vi "When Read U32.vi"(0 "error out":errorcluster, 1 "value":u32, 11 "Configuration In":refnum<class "Mock Configuration.lvclass">) -> (3 "Configuration Out":refnum<class "Mock Configuration.lvclass">)   [LabVIEW 2020, in "Mock Configuration.lvclass"]
doc: "High-level function for reading configuration file data from process class. If the specified key is not present, it is added with the configured default value."
uses:
  Mock Configuration.lvclass
  Mock Configuration.lvclass/Mock Configuration.ctl
  <vilib>/Astemes/LMock/Mock.lvclass
  C:/Program Files (x86)/National Instruments/LabVIEW 2020/vi.lib/Astemes/LMock/Mock.lvclass
  C:/git/danfoss-excel-report-teststand-plugin/tests/Mock Configuration/Mock Configuration.lvclass
  C:/git/danfoss-excel-report-teststand-plugin/source/TestStand Public/Components/Models/ModelPlugin/Astemes_CSVReportGenerator/Configuration/Configuration.lvclass
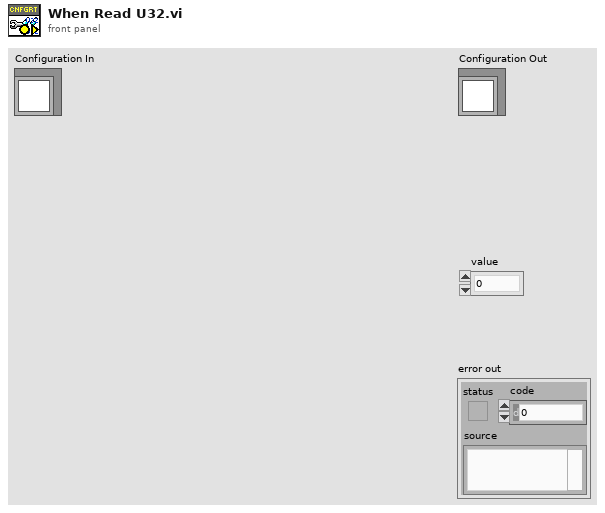
[diagram p1: front panel]
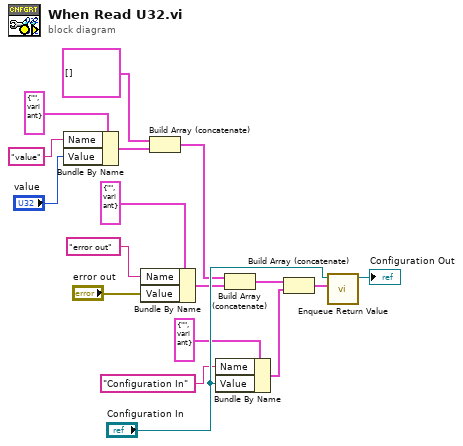
[diagram p0: block diagram]
diagram:
  n1 = Bundle By Name(cluster=cluster{"Name":string, "Value":variant} {"Name"="", "Value"=variant} ("element"), "Name"="value", "Value"="value") -> (w5:cluster{"Name":string, "Value":variant})
  n2 = Bundle By Name(cluster=cluster{"Name":string, "Value":variant} {"Name"="", "Value"=variant} ("element"), "Name"="error out", "Value"="error out") -> (w3:cluster{"Name":string, "Value":variant})
  n3 = Build Array (concatenate)(cluster{"Name":string, "Value":variant}[] [] ("Control Values"), w5) -> (w10:cluster{"Name":string, "Value":variant}[])
  n4 = Bundle By Name(cluster=cluster{"Name":string, "Value":variant} {"Name"="", "Value"=variant} ("element"), "Name"="Configuration In", "Value"="Configuration In") -> (w1:cluster{"Name":string, "Value":variant})
  n5 = Build Array (concatenate)(w10, w3) -> (w13:cluster{"Name":string, "Value":variant}[])
  n6 = Build Array (concatenate)(w13, w1) -> (w15:cluster{"Name":string, "Value":variant}[])
  n7 = call <vilib>:"Enqueue Return Value.vi"("Indicator Values"=w15, "Mock In"="Configuration In") -> ("Mock Out"=→"Configuration Out":refnum<class "Mock Configuration.lvclass">)  [unwired: 8 in, 1 out]
